vi "REC RATE.vi"(0 "System no.":i32=1 min=1 max=4 step=1, 2 "RecorderIDs":string[](array[string]), 3 "Recording rate":i32[](array[numeric]), 5 "error in":errorcluster) -> (19 "error out":errorcluster)   [LabVIEW 2020]
doc: "REC RATE (Configure Recording Rate)\n\nDescription\nConfigures a data recorder for recording:\nSets the recording rate.\nA data recorder can only be configured when it is in the state \"CFG\", see the state diagram for \nthe data recorder (p. 110). The state of the data recorder can be queried with REC? STATE\n(p. 47). \n\nFormat \nREC RATE <RecorderID> <RecordingRate>\n\nArguments\n<RecorderID>\nData recorder, whose recording rate is to be set; to be specified as alias (p. 94) \nThe available data recorders can be queried with USG? SYS (p. 80). \nPossible values: REC_1 to RECn, where n = number of data recorders in the controller\n<RecordingRate>\nRecording rate; given as the number of servo cycles\nThe recording rate specifies after how many servo cycles the next data point is recorded. The \nhigher the recording rate, the longer the recording takes.\nPossible values: UINT >= 1\n\nResponse\nnone\n\nExample\n>>REC? RATE\n<<REC_1=10\n<<REC_2=10\n>>REC RATE REC_1 1\n>>ERR?\n<<0 - (error 0 - \"No error\")\n>>REC? RATE\n<<REC_1=1\n<<REC_2=10\n\nNotes\nThe recording rate influences the duration of the recording. Example:\nThe servo cycle time of the controller is tS = 50 µs.\nAt a recording rate of r = 5 the time between two data points is td = r • tS = 250 µs.\nFor further details, see \"Data Recorder - GCS 3.0\" (p. 107). \n\nUser command level\nUSR"
panel:
  # "REC RATE (Configure Recording Rate)\n\nConfigures a data recorder for recording:\nSets the recording rate.\nA data recorder can only be configured when it is in the state \"CFG\", see the state diagram for  the data recorder. The state of the data recorder can be queried with REC? STATE."
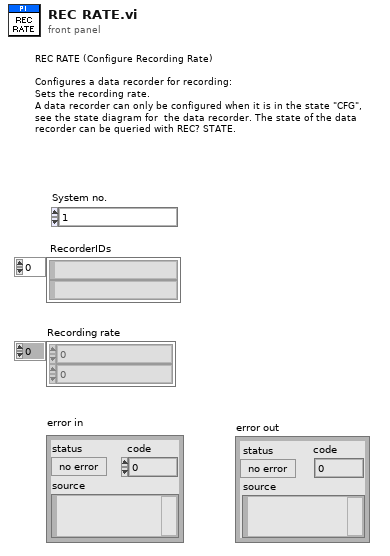
[diagram p1: front panel]
types:
  T1 = typedef "Syntax.ctl" = enum16{"GCS 1.0", "GCS 2.0", "GCS 3.0"}
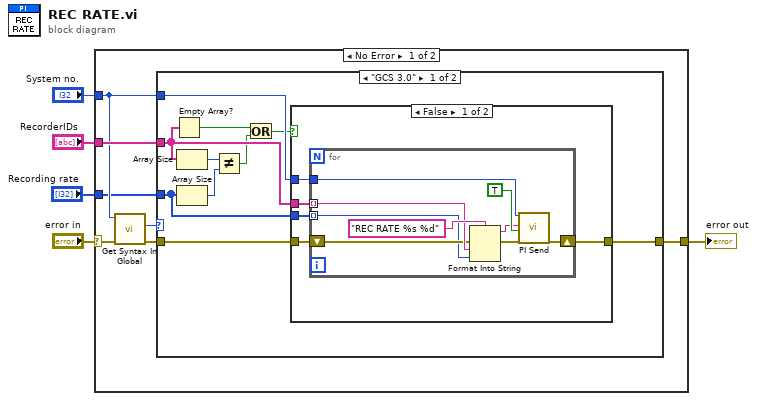
[diagram p0: block diagram]
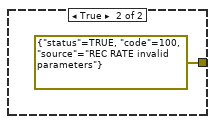
[diagram p2: hidden frame]
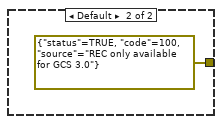
[diagram p3: hidden frame]
diagram:
  n1 = case shown="No Error" "error in" {
    selector: "error in" -> [w12 w39]
    tunnel: [w9 w39] -> w2
    tunnel: "RecorderIDs" -> [w8 _]
    tunnel: "System no." -> [w7 _]
    tunnel: "Recording rate" -> [w6 _]
    frame No Error {
      n2 = call "Get Syntax In Global.vi"("error in"=w12, "System no."=w7) -> ("error out"=w10:errorcluster, "Syntax"=w11:T1)  [unwired: 8 in]
      n3 = case shown="\"GCS 3.0\"" w11 {
        tunnel: w10 -> [w22 _]
        tunnel: [w21 errorcluster {"status"=TRUE, "code"=100, "source"="REC only available for GCS 3.0"} ("error out")] -> w9
        tunnel: w8 -> [w19 _]
        tunnel: w7 -> [w20 _]
        tunnel: w6 -> [w18 _]
        frame "GCS 3.0" {
          n4 = Empty Array?(array=w19) -> (empty?=w15:bool)
          n5 = Array Size(array=w19) -> (size(s)=w16:i32)
          n6 = Array Size(array=w18) -> (size(s)=w17:i32)
          n7 = Not Equal?(x=w16, y=w17) -> (x != y?=w14:bool)
          n8 = Or(x=w15, y=w14) -> (x .or. y?=w13:bool)
          n9 = case shown="False" w13 {
            tunnel: w19 -> [w27 _]
            tunnel: w18 -> [w26 _]
            tunnel: w22 -> [w25 _]
            tunnel: [w24 errorcluster {"status"=TRUE, "code"=100, "source"="REC RATE invalid parameters"} ("error out")] -> w21
            tunnel: w20 -> [w23 _]
            frame False {
              n10 = for {
                tunnel: w27 -> [w35] mode=indexing
                tunnel: w26 -> [w28] mode=indexing
                shift-right: [w32] -> w24
                shift-left: w25 -> [w34]
                tunnel: w23 -> [w29]
                n11 = Format Into String(format string="REC RATE %s %d", error in=w34, w35, w28) -> (resulting string=w30:string, error out=w33:errorcluster)  [unwired: 1 in]
                n12 = call "PI Send.vi"("System no."=w29, "String to send"=w30, "Attach termination char.?"=TRUE, "error in"=w33) -> ("error out"=w32:errorcluster)  [unwired: 2 in, 13 out]
              }
            }
            frame True {
            }
          }
        }
        frame Default {
        }
      }
    }
    frame Error {
    }
  }
  "error out" <- w2
